vi "Run Tests.vi"(8 "error in (no error)":errorcluster, 10 "Tests to Run":refnum<class "_test class base.lvclass">[](array[class]), 11 "object in":refnum<class "Tesla Factory Tester.lvclass">) -> (0 "error out":errorcluster, 3 "object out":refnum<class "Tesla Factory Tester.lvclass">)   [LabVIEW 2013, in "Tesla Factory Tester.lvlib" / "Tesla Factory Tester.lvclass"]
uses:
  Tesla Factory Tester.lvclass
  _test class base/_test class base_Actor/_test class base.lvclass
  <vilib>/ActorFramework/Actor/Actor.lvclass/Actor.ctl
  <vilib>/ActorFramework/Message Enqueuer/Message Enqueuer.lvclass/Message Enqueuer.ctl
  Messages/Update Status String_Msg/Update Status String_Msg.lvclass/Update Status String_Msg.ctl
  Tesla Factory Tester.lvclass/Tesla Factory Tester.ctl
  <vilib>/ActorFramework/Message Enqueuer/Init from Existing Queue.vi
  <vilib>/ActorFramework/Message Enqueuer/Enqueue.vi
  <vilib>/ActorFramework/Message Priority Queue/Priority Enqueue.vi
  <vilib>/ActorFramework/Message Enqueuer/Message Enqueuer.lvclass
  Messages/Update Status String_Msg/Update Status String_Msg.lvclass
  <vilib>/ActorFramework/Actor/Actor.lvclass
panel:
  in  "Run Concurrently?(T)":bool=TRUE
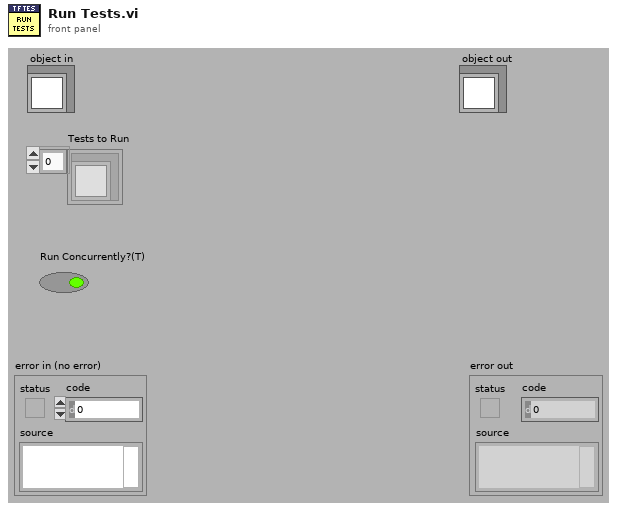
[diagram p1: front panel]
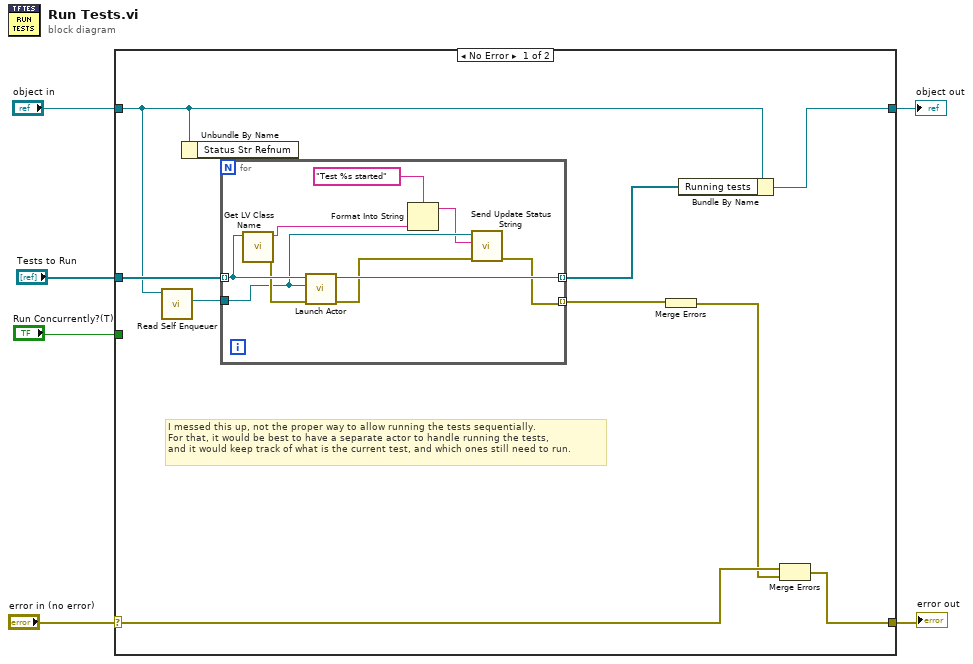
[diagram p0: block diagram]
diagram:
  n1 = case shown="No Error" "error in (no error)" {
    selector: "error in (no error)" -> [w13 w26]
    tunnel: [w11 w26] -> w5
    tunnel: [w7 w25] -> w3
    tunnel: "object in" -> [w9 w25]
    tunnel: "Run Concurrently?(T)" -> [_ _]
    tunnel: "Tests to Run" -> [w15 _]
    frame No Error {
      # "I messed this up, not the proper way to allow running the tests sequentially.\nFor that, it would be best to have a separate actor to handle running the tests,\nand it would keep track of what is the current test, and which ones still need to run."
      n2 = call <vilib>:"Read Self Enqueuer.vi"("Actor"=w9) -> ("Self Enqueuer"=w14:refnum<class "Message Enqueuer.lvclass">)  [unwired: 10 in]
      n3 = Unbundle By Name(w9) -> ()  [unwired: 1 out]
      n4 = for {
        tunnel: w15 -> [w23] mode=indexing
        tunnel: w14 -> [w20]
        tunnel: [w19] -> w10 mode=indexing
        tunnel: [w24] -> w8 mode=indexing
        n5 = call <vilib>:"Get LV Class Name.vi"("object"=w23) -> ("error out"=w22:errorcluster, "class name"=w16:string)  [unwired: 9 in]
        n6 = call <vilib>:"Launch Actor.vi"("error in (no error)"=w22, "Actor-to-Caller Enqueuer"=w20, "Actor"=w23) -> ("error out"=w21:errorcluster, "Caller-To-Actor Enqueuer"=w24:refnum<class "Message Enqueuer.lvclass">)  [unwired: 7 in]
        n7 = Format Into String(format string="Test %s started", w16) -> (resulting string=w17:string)  [unwired: 2 in, 1 out]
        n8 = call "Send Update Status String.vi"("error in (no error)"=w21, "Append this string"=w17, "Message Enqueuer"=w20) -> ("error out"=w19:errorcluster)  [unwired: 7 in, 1 out]
      }
      n9 = Merge Errors(w10) -> (w12:errorcluster)
      n10 = Bundle By Name(cluster=w9, "Running tests"=w8) -> (w7:refnum<class "Tesla Factory Tester.lvclass">)
      n11 = Merge Errors(w13, w12) -> (w11:errorcluster)
    }
    frame Error {
    }
  }
  "error out" <- w5
  "object out" <- w3
